vi "Init Test Object.vi"(8 "error in (no error)":errorcluster, 10 "Int (0)":i32) -> (0 "error out":errorcluster, 3 "Numeric out":refnum<class "Numeric Test Object.lvclass">)   [LabVIEW 2009]
doc: "Creates a numeric test object and initializes all values."
uses:
  Numeric Test Object/Numeric Test Object.lvclass
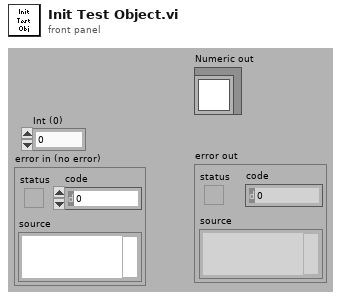
[diagram p1: front panel]
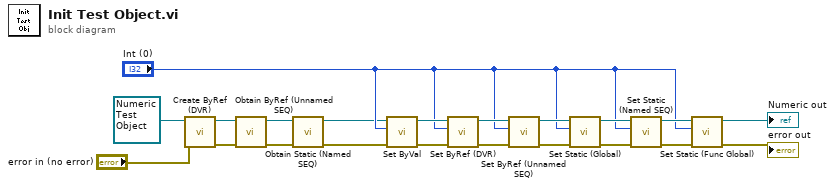
[diagram p0: block diagram]
diagram:
  n1 = call-dynamic "Create ByRef (DVR).vi"("error in (no error)"="error in (no error)", "Numeric in"=refnum<class "Numeric Test Object.lvclass"> refnum ("Numeric")) -> ("error out"=w19:errorcluster, "Numeric out"=w20:refnum<class "Numeric Test Object.lvclass">)  [unwired: 8 in]
  n2 = call-dynamic "Obtain ByRef (Unnamed SEQ).vi"("error in (no error)"=w19, "Numeric in"=w20) -> ("error out"=w4:errorcluster, "Numeric out"=w7:refnum<class "Numeric Test Object.lvclass">)  [unwired: 8 in]
  n3 = call-dynamic "Obtain Static (Named SEQ).vi"("error in (no error)"=w4, "Numeric in"=w7) -> ("error out"=w5:errorcluster, "Numeric out"=w6:refnum<class "Numeric Test Object.lvclass">)  [unwired: 8 in]
  n4 = call-dynamic "Set ByVal.vi"("error in (no error)"=w5, "Int"="Int (0)", "Numeric in"=w6) -> ("error out"=w12:errorcluster, "Numeric out"=w18:refnum<class "Numeric Test Object.lvclass">)  [unwired: 7 in]
  n5 = call-dynamic "Set ByRef (DVR).vi"("error in (no error)"=w12, "Int"="Int (0)", "Numeric in"=w18) -> ("error out"=w11:errorcluster, "Numeric out"=w17:refnum<class "Numeric Test Object.lvclass">)  [unwired: 7 in]
  n6 = call-dynamic "Set ByRef (Unnamed SEQ).vi"("error in (no error)"=w11, "Int"="Int (0)", "Numeric in"=w17) -> ("error out"=w10:errorcluster, "Numeric out"=w16:refnum<class "Numeric Test Object.lvclass">)  [unwired: 7 in]
  n7 = call-dynamic "Set Static (Global).vi"("error in (no error)"=w10, "Int"="Int (0)", "Numeric in"=w16) -> ("error out"=w9:errorcluster, "Numeric out"=w15:refnum<class "Numeric Test Object.lvclass">)  [unwired: 7 in]
  n8 = call-dynamic "Set Static (Named SEQ).vi"("error in (no error)"=w9, "Int"="Int (0)", "Numeric in"=w15) -> ("error out"=w8:errorcluster, "Numeric out"=w14:refnum<class "Numeric Test Object.lvclass">)  [unwired: 7 in]
  n9 = call-dynamic "Set Static (Func Global).vi"("error in (no error)"=w8, "Int"="Int (0)", "Numeric in"=w14) -> ("error out"=→"error out":errorcluster, "Numeric out"=→"Numeric out":refnum<class "Numeric Test Object.lvclass">)  [unwired: 7 in]
